vi "Air MFR sw 3.vi"(8 "Increment":dbl, 10 "C_air":dbl, 11 "Flow rate":dbl) -> (3 "Air MFR":dbl)   [LabVIEW 2014]
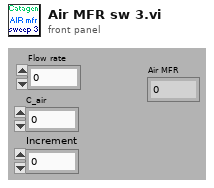
[diagram p1: front panel]
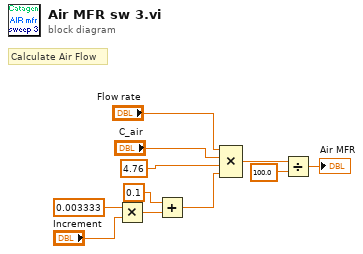
[diagram p0: block diagram]
diagram:
  # "Calculate Air Flow"
  n1 = Multiply(x=0.003333, y="Increment") -> (x*y=w7:dbl)
  n2 = Add(x=0.1, y=w7) -> (x+y=w1:dbl)
  n3 = Compound Arithmetic op=MULTIPLY("Flow rate", "C_air", 4.76, w1) -> (w9:dbl)
  n4 = Divide(x=w9, y=100.0) -> (x/y=→"Air MFR":dbl)
